vi "fetch_selection_node_reference.vi"(8 "error in":errorcluster, 11 "vs_tree_control in":refnum<class "vs_tree_control.lvclass">) -> (0 "error out":errorcluster, 2 "Selected Node":refnum<k24>, 3 "vs_tree_control out":refnum<class "vs_tree_control.lvclass">)   [LabVIEW 2020, in "vs_tree_control.lvclass"]
uses:
  vs_tree_control.lvclass
  NationalInstruments.VeriStand.SystemStorage
  NationalInstruments.VeriStand.SystemStorageUI
  NationalInstruments.VeriStand.SystemDefinitionAPI
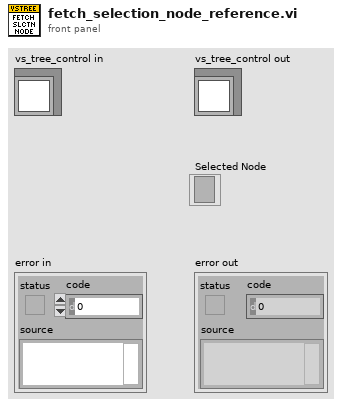
[diagram p1: front panel]
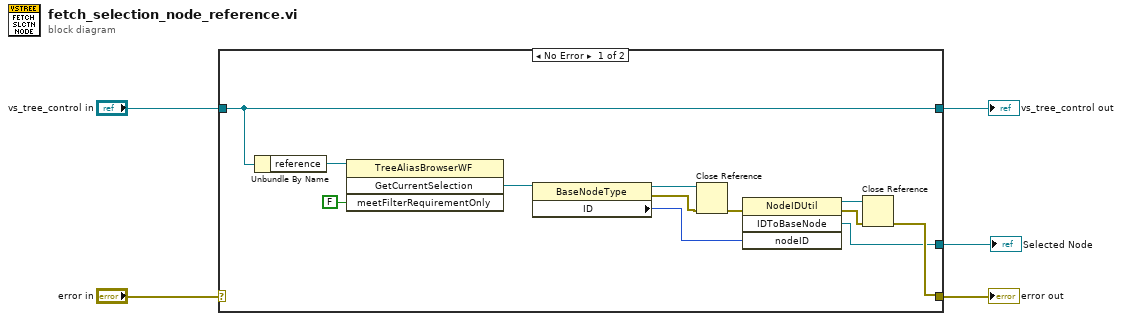
[diagram p0: block diagram]
diagram:
  n1 = case shown="No Error" "error in" {
    selector: "error in" -> [_ w19]
    tunnel: [w7 w19] -> w4
    tunnel: [w17 w18] -> w2
    tunnel: "vs_tree_control in" -> [w17 w18]
    tunnel: [w6 _] -> w1
    frame No Error {
      n2 = Unbundle By Name(w17) -> ("reference"=w16:refnum<k24>)
      n3 = invoke class="TreeAliasBrowserWF" method="GetCurrentSelection"(reference=w16, "meetFilterRequirementOnly"=FALSE) -> ("GetCurrentSelection"=w13:refnum<k24>)  [unwired: 2 in, 3 out]
      n4 = property class="BaseNodeType"(reference=w13) -> (reference out=w12:refnum<k24>, error out=w11:errorcluster, "ID"=w14:u64)  [unwired: 1 in]
      n5 = Close Reference(reference=w12, error in (no error)=w11) -> (error out=w10:errorcluster)
      n6 = invoke class="NodeIDUtil" method="IDToBaseNode"(error in=w10, "nodeID"=w14) -> (reference out=w9:refnum<k24>, error out=w8:errorcluster, "IDToBaseNode"=w6:refnum<k24>)  [unwired: 2 in, 1 out]
      n7 = Close Reference(reference=w9, error in (no error)=w8) -> (error out=w7:errorcluster)
    }
    frame Error {
    }
  }
  "error out" <- w4
  "vs_tree_control out" <- w2
  "Selected Node" <- w1
